vi "Configure Format Border.vi"(8 "error in (no error)":errorcluster, 10 "Byte Order (0: Normal)":i32(ring) items=["Normal", "Swapped"], 11 "VISA resource name":refnum<visa-resource-name>) -> (0 "error out":errorcluster, 3 "VISA resource name out":refnum<visa-resource-name>)   [LabVIEW 2016, in "Agilent 3352X Series.lvlib"]
doc: "Selects the byte order which will be used to make binary data point transfers in the block mode.\n\n<B>Note</B>:\nThis VI does not check the instrument status."
uses:
  Agilent 3352X Series.lvlib
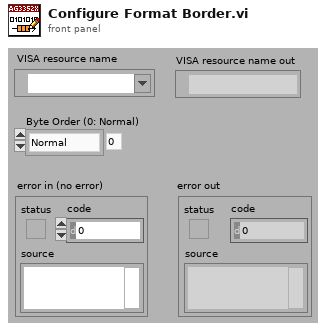
[diagram p1: front panel]
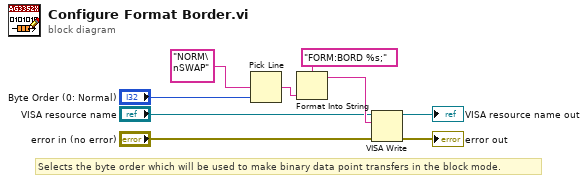
[diagram p0: block diagram]
diagram:
  # "Selects the byte order which will be used to make binary data point transfers in the block mode."
  n1 = Pick Line(multi-line string="NORM\nSWAP", line index="Byte Order (0: Normal)") -> (output string=w1:string)  [unwired: 1 out]
  n2 = Format Into String(format string="FORM:BORD %s;", w1) -> (resulting string=w8:string)  [unwired: 2 in, 1 out]
  n3 = VISA Write(VISA resource name="VISA resource name", write buffer=w8, error in (no error)="error in (no error)") -> (VISA resource name out=→"VISA resource name out":refnum<visa-resource-name>, error out=→"error out":errorcluster)  [unwired: 1 out]
